vi "Get Checkbox Row At Coordinates.vi"(8 "error in (no error)":errorcluster, 10 "Coords":T2, 11 "MCListbox with Checkboxes in":refnum<class "MCListbox with Checkboxes.lvclass">) -> (0 "error out":errorcluster, 1 "Index":i32, 2 "In Check?":bool, 3 "MCListbox with Checkboxes out":refnum<class "MCListbox with Checkboxes.lvclass">, 4 "CellPosition":T1, 6 "In Bounds?":bool)   [LabVIEW 2016, in "MCListbox with Checkboxes.lvclass"]
uses:
  MCListbox with Checkboxes.lvclass
  <vilib>/Utility/miscctls.llb/LVPositionTypeDef.ctl
  <vilib>/Utility/miscctls.llb/LVRowAndColumnTypeDef.ctl
  MCListbox with Checkboxes.lvclass/MCListbox with Checkboxes.ctl
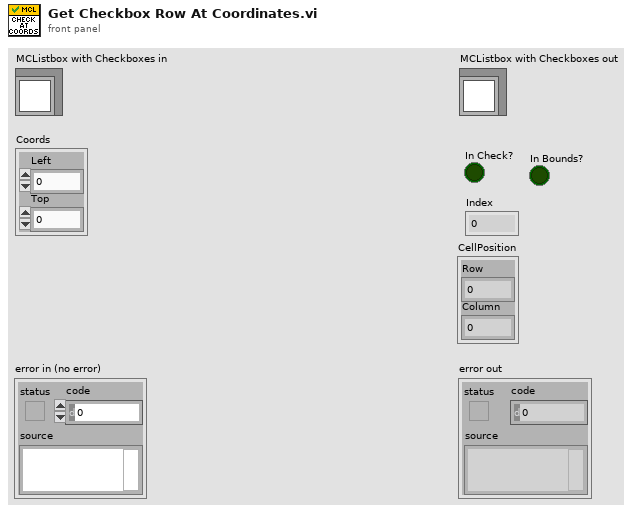
[diagram p1: front panel]
types:
  T1 = typedef "LVRowAndColumnTypeDef.ctl" = cluster{"Row":i32, "Column":i32}
  T2 = typedef "LVPositionTypeDef.ctl" = cluster{"Left":i32, "Top":i32}
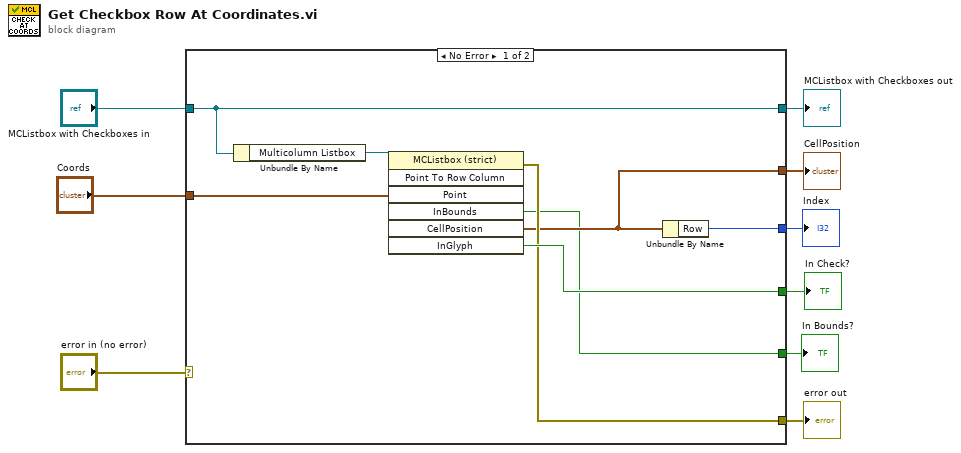
[diagram p0: block diagram]
diagram:
  n1 = case shown="No Error" "error in (no error)" {
    selector: "error in (no error)" -> [_ w19]
    tunnel: [w12 w19] -> w8
    tunnel: [w17 w18] -> w6
    tunnel: "MCListbox with Checkboxes in" -> [w17 w18]
    tunnel: "Coords" -> [w15 _]
    tunnel: [w14 _] -> w4
    tunnel: [w13 _] -> w3
    tunnel: [w11 _] -> w2
    tunnel: [w10 _] -> w1
    frame No Error {
      n2 = Unbundle By Name(w17) -> ("Multicolumn Listbox"=w16:refnum<vi>)
      n3 = invoke class="MCListbox (strict)" method="Point To Row Column"(reference=w16, "Point"=w15) -> (error out=w12:errorcluster, "InBounds"=w10:bool, "CellPosition"=w11:T1, "InGlyph"=w13:bool)  [unwired: 5 in, 3 out]
      n4 = Unbundle By Name(w11) -> ("Row"=w14:i32)
    }
    frame Error {
    }
  }
  "error out" <- w8
  "MCListbox with Checkboxes out" <- w6
  "Index" <- w4
  "In Check?" <- w3
  "CellPosition" <- w2
  "In Bounds?" <- w1
